vi "GetDataType.vi"(8 "error in":errorcluster, 11 "Tunnel in":refnum<class "FlatSequenceOuterTunnel.lvclass">) -> (0 "error out":errorcluster, 2 "Data Type":variant, 3 "Tunnel out":refnum<class "FlatSequenceOuterTunnel.lvclass">)   [LabVIEW 2014, in "FlatSequenceOuterTunnel.lvclass"]
uses:
  FlatSequenceOuterTunnel.lvclass
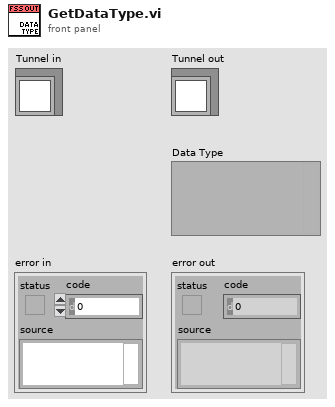
[diagram p1: front panel]
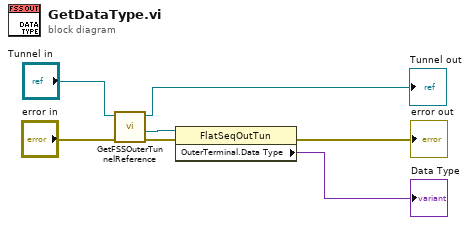
[diagram p0: block diagram]
diagram:
  n1 = call "GetFSSOuterTunnelReference.vi"("error in"="error in", "Tunnel in"="Tunnel in") -> ("error out"=w6:errorcluster, "reference out"=w7:refnum<vi>, "Tunnel out"=→"Tunnel out":refnum<class "FlatSequenceOuterTunnel.lvclass">)  [unwired: 7 in]
  n2 = property class="FlatSeqOutTun"(reference=w7, error in=w6) -> (error out=→"error out":errorcluster, "OuterTerminal.Data Type"=→"Data Type":variant)  [unwired: 1 out]
